vi "zenith_angle.vi"(1 "Time (hour of day)":dbl, 2 "Day of Year (day)":dbl, 3 "Latitude (rad, +:N, -:S)":dbl) -> (0 "Zenith angle (rad)":dbl)   [LabVIEW 2012]
panel:
  out "Zenith angle (¼)":dbl
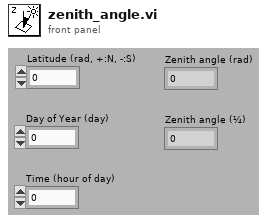
[diagram p1: front panel]
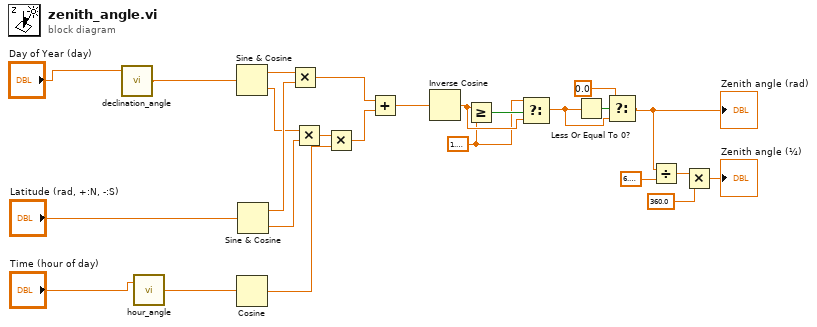
[diagram p0: block diagram]
diagram:
  w8 = 1.5707963267948966
  n1 = call "declination_angle.vi"("Day of Year (day)"="Day of Year (day)") -> ("Declination (rad)"=w2:dbl)  [unwired: 2 in]
  n2 = call "hour_angle.vi"("Time (hour of day since midnight)"="Time (hour of day)") -> ("Hour angle h (rad)"=w16:dbl)  [unwired: 1 in]
  n3 = Sine & Cosine(0:w2) -> (1:w25:dbl, 2:w22:dbl)
  n4 = Cosine(x=w16) -> (cos(x)=w18:dbl)
  n5 = Sine & Cosine(0:"Latitude (rad, +:N, -:S)") -> (1:w24:dbl, 2:w19:dbl)
  n6 = Multiply(x=w25, y=w24) -> (x*y=w23:dbl)
  n7 = Multiply(x=w22, y=w19) -> (x*y=w21:dbl)
  n8 = Multiply(x=w21, y=w18) -> (x*y=w20:dbl)
  n9 = Add(x=w23, y=w20) -> (x+y=w15:dbl)
  n10 = Inverse Cosine(1:w15) -> (0:w9:dbl)
  n11 = Greater Or Equal?(x=w9, y=w8) -> (x >= y?=w10:bool)
  n12 = Select(t=w8, s=w10, f=w9) -> (s? t:f=w6:dbl)
  n13 = Less Or Equal To 0?(x=w6) -> (x <= 0?=w7:bool)
  n14 = Select(t=0.0, s=w7, f=w6) -> (s? t:f=w5:dbl)
  "Zenith angle (rad)" <- w5
  n15 = Divide(x=w5, y=6.283185307179586) -> (x/y=w13:dbl)
  n16 = Multiply(x=w13, y=360.0) -> (x*y=→"Zenith angle (¼)":dbl)
